vi "SW_Add_Reward_Condition.vi"(8 "error in (no error)":T11, 9 "Main Tree Control in":refnum<vi>, 10 "Calibration parameters":T9={"Timing calibration sw/hw"=1.0, "True FPS"=80.0, "True frame time, s"=0.0125, "Disp. calibration info"=[]} {"True frame time, s" format="%.10g"; "Disp. calibration info"."Speed, µl per ms" format="%.3g"; "True FPS" format="%.10g"; "Timing calibration sw/hw" format="%.10g"}, 11 "Array of conditions in":T8 {"Response"."TTL pulse length, ms" min=0.0 max=10000.0 step=10.0; "Specifier(s)"."Validity criteria(s)"."Validity value" min=0.0 step=0.1 format="%.2g"; "Specifier(s)"."Value" step=1.0 format="%#.2g"}) -> (0 "error out":T11, 3 "Array of conditions out":T8 {"Response"."TTL pulse length, ms" min=0.0 max=10000.0 step=10.0; "Specifier(s)"."Validity criteria(s)"."Validity value" min=0.0 step=0.1 format="%.2g"; "Specifier(s)"."Value" step=1.0 format="%#.2g"})   [LabVIEW 2018, in "Tracker.lvlib"]
uses:
  Tracker.lvlib
  Controls/CTL_Conditions_Array.ctl
  Controls/CTL_Conditions_Cluster.ctl
  Controls/CTL_Condition_type.ctl
  Controls/CTL_Comparison_type.ctl
  Controls/CTL_Validity_check_criteria.ctl
  Controls/CTL_Condition_response_type.ctl
  Controls/CTL_Calibration_parameters.ctl
  Controls/CTL_Dispenser_calibration_info.ctl
  <vilib>/Utility/miscctls.llb/LVPointTypeDef.ctl
panel:
  in  "Save SubCondition":bool
  out "Validity criteria(s)":T2(array[cluster])
  out "Subcondition":T3={"Enabled"=FALSE, "Name"="", "Specifier(s)"=[], "Response"={"Response type"=enum."Air puff", "TTL port"=enum."TTL", "TTL pulse length, ms"=0.0}} caption="Condition" {"Specifier(s)"."Validity criteria(s)"."Validity value" min=0.0 step=0.1 format="%.2g"; "Specifier(s)"."Value" step=1.0 format="%#.2g"}
  in  "TTL pulse length":dbl caption="Disp. volume, ul"
  in  "TTL port":enum16{"TTL"}(ring)
  in  "Response type":T6=enum."Air puff"
  in  "Valid for, units":dbl caption="Has been True for, units" format="%.2g"
  in  "Validity Enabled":bool caption="Enabled"
  in  "SC. Validity Criteria":T1 caption="Validity Criteria"
  in  "Compare against":dbl
  in  "Comparison type":T5
  in  "SubCondition type":T4
  in  "Specifier Enabled":bool caption="Enabled"
  in  "Subcondition #":i32(slide)=5 min=1 max=5 step=1 scale=5.0..1.0
  in  "Specifier(s)":T7(array[cluster])
  in  "C. Name":string caption="Condition Name"
  out "N conditions":i32
  in  "C. Enabled":bool caption="Enabled"
  out "Selected SubCondition":string
  out "Selected Condition":string
  out "Review changes before save":string(tree) caption="Reward and stimulation out"
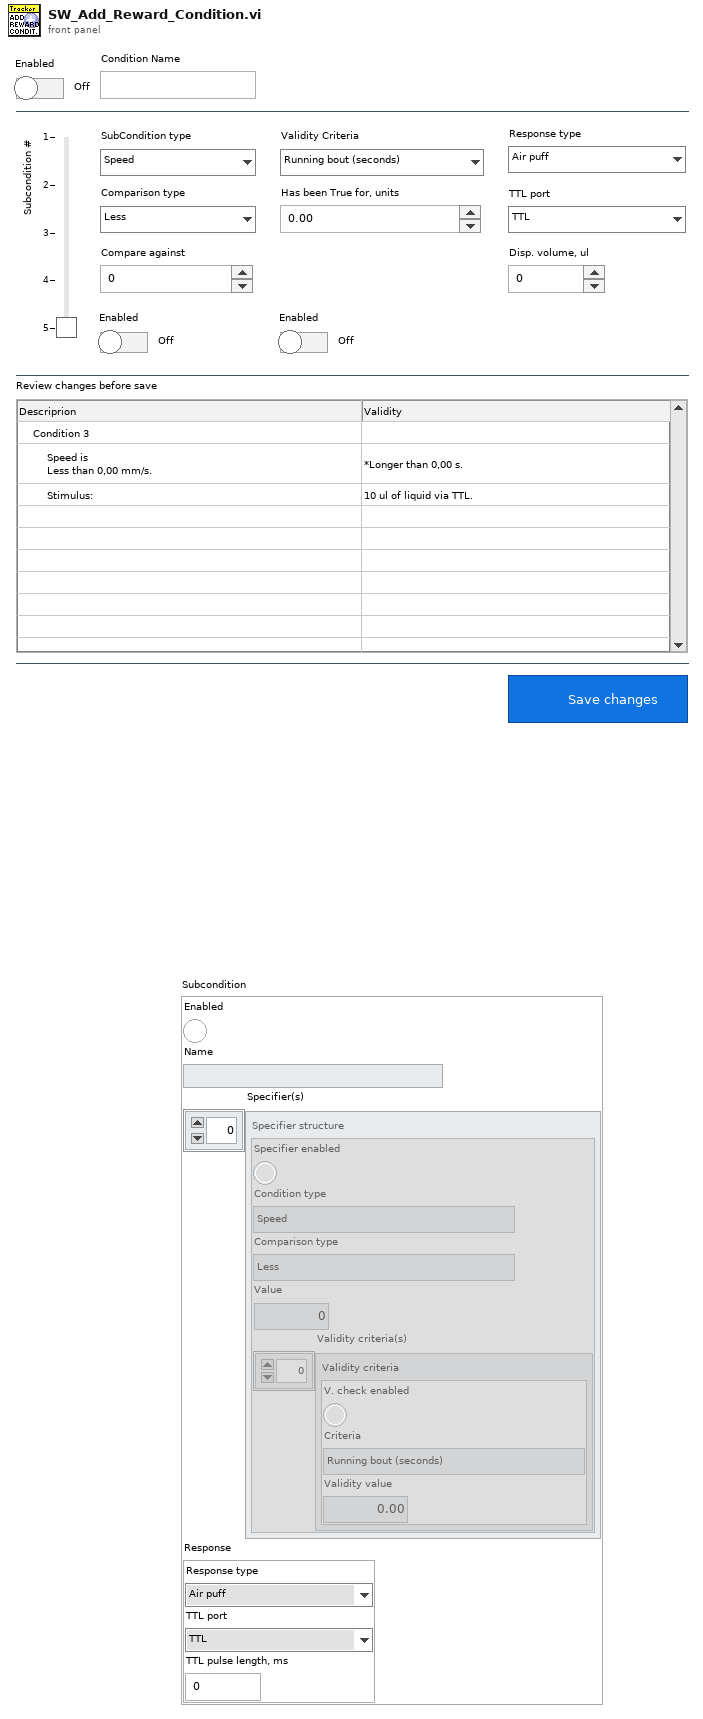
[diagram p1: front panel]
types:
  T1 = typedef "Tracker.lvlib/CTL_Validity_check_criteria.ctl" = enum16{"Running bout (seconds)", "Running bout (meters)"}
  T2 = cluster{"V. check enabled":bool, "Criteria":T1, "Validity value":dbl}[]
  T3 = typedef "Tracker.lvlib/CTL_Conditions_Cluster.ctl" = cluster{"Enabled":bool, "Name":string, "Specifier(s)":cluster{"Specifier enabled":bool, "Condition type":T4, "Comparison type":T5, "Value":dbl, "Validity criteria(s)":cluster{"V. check enabled":bool, "Criteria":T1, "Validity value":dbl}[]}[], "Response":cluster{"Response type":T6, "TTL port":enum16{"TTL"}, "TTL pulse length, ms":dbl}}
  T4 = typedef "Tracker.lvlib/CTL_Condition_type.ctl" = enum16{"Speed", "Zone", "Angle to wall"}
  T5 = typedef "Tracker.lvlib/CTL_Comparison_type.ctl" = enum16{"Less", "Less or Equal", "Equal", "Greater or Equal", "Greater", "Not Equal"}
  T6 = typedef "Tracker.lvlib/CTL_Condition_response_type.ctl" = enum16{"None", "Air puff", "Liquid reward"}
  T7 = cluster{"Specifier enabled":bool, "Condition type":T4, "Comparison type":T5, "Value":dbl, "Validity criteria(s)":cluster{"V. check enabled":bool, "Criteria":T1, "Validity value":dbl}[]}[]
  T8 = typedef "Tracker.lvlib/CTL_Conditions_Array.ctl" = T3[]
  T9 = typedef "Tracker.lvlib/CTL_Calibration_parameters.ctl" = cluster{"Timing calibration sw/hw":dbl, "True FPS":dbl, "True frame time, s":dbl, "Disp. calibration info":T10}
  T10 = typedef "Tracker.lvlib/CTL_Dispenser_calibration_info.ctl" = cluster{"Channel":u8, "Speed, µl per ms":dbl}[]
  T11 = cluster{"Boolean Round":bool, "code":i32, "source":string}
  T12 = typedef "LVPointTypeDef.ctl" = cluster{"Horizontal":i16, "Vertical":i16}
  T13 = cluster{"Response type":T6, "TTL port":enum16{"TTL"}, "TTL pulse length, ms":dbl}
  T14 = cluster{"Specifier enabled":bool, "Condition type":T4, "Comparison type":T5, "Value":dbl, "Validity criteria(s)":cluster{"V. check enabled":bool, "Criteria":T1, "Validity value":dbl}[]}
  T15 = cluster{"V. check enabled":bool, "Criteria":T1, "Validity value":dbl}
  T16 = cluster{"Validity Enabled":bool, "SC. Validity Criteria":T1, "Valid for, units":dbl}
  T17 = cluster{"Response type":T6, "TTL port":enum16{"TTL"}, "TTL pulse length, ms out":dbl}
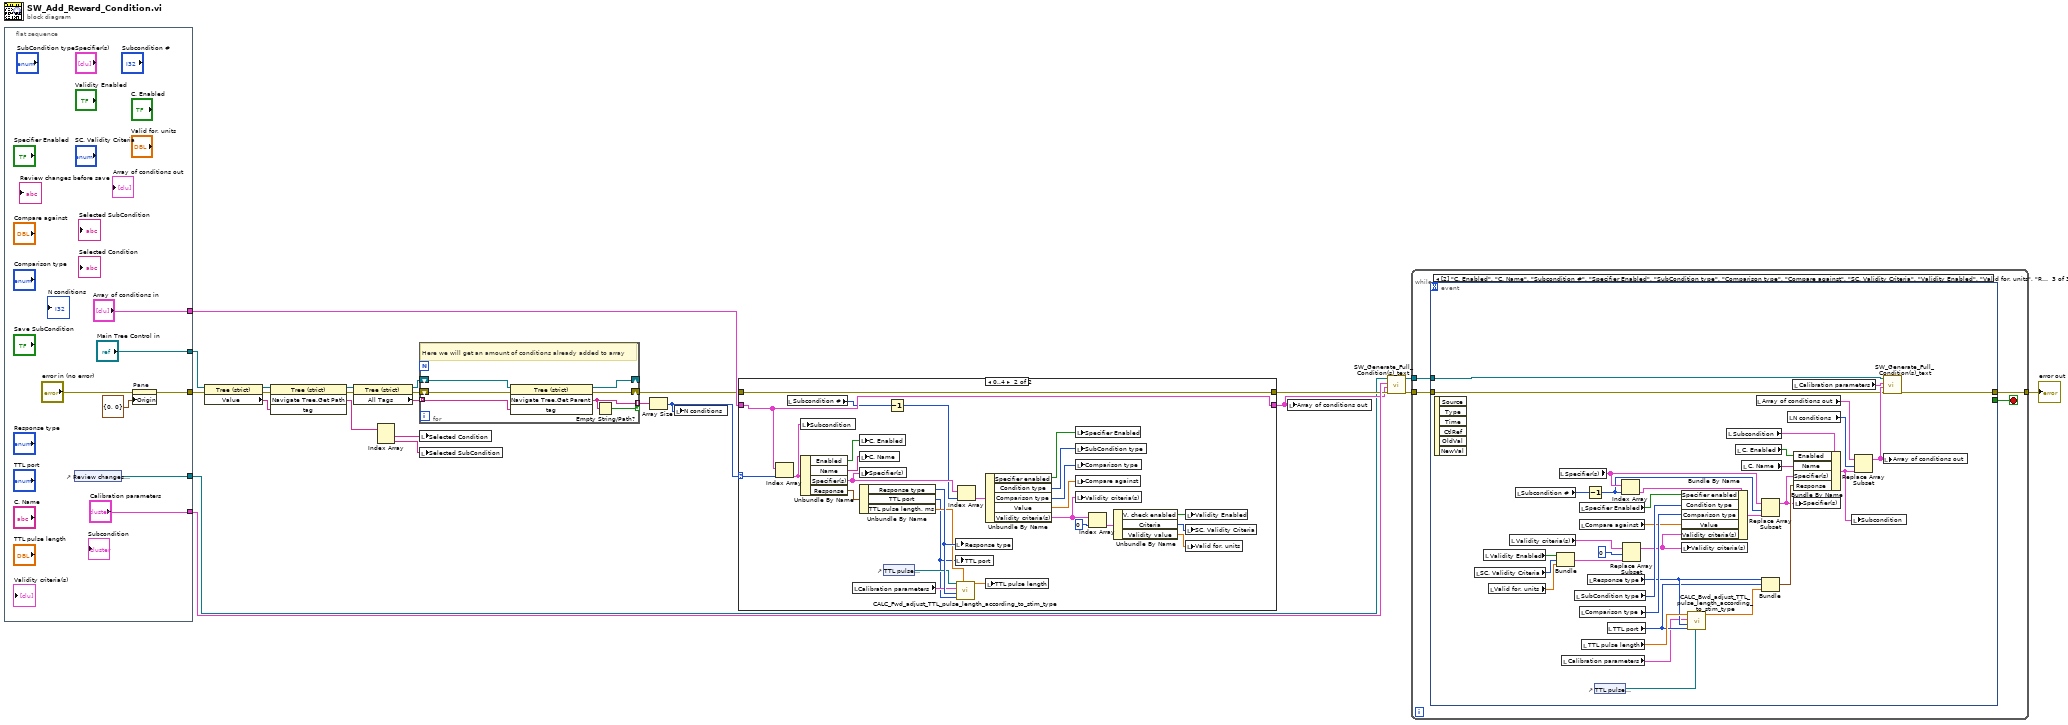
[diagram p0: block diagram]
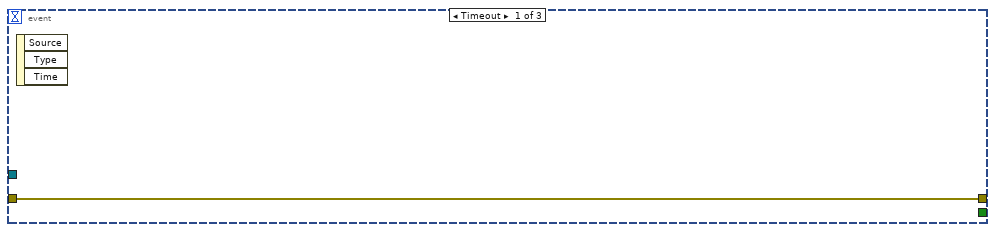
[diagram p2: hidden frame]
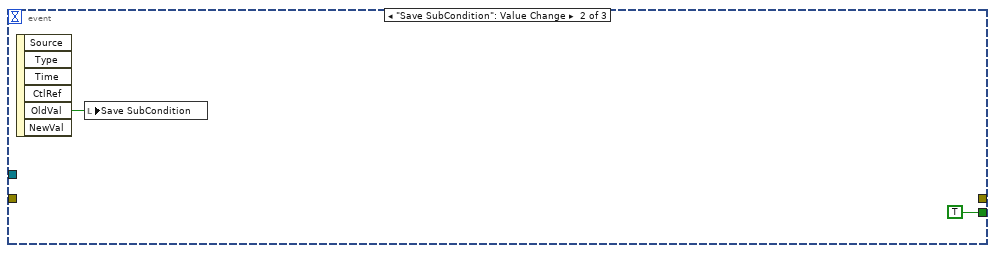
[diagram p3: hidden frame]
diagram:
  n1 = flat-sequence {
    tunnel: [w31] -> w13
    tunnel: [w28] -> w2
    tunnel: ["Main Tree Control in"] -> w24
    tunnel: ["Array of conditions in"] -> w15
    tunnel: ["Calibration parameters"] -> w14
    frame #0 {
      n2 = control-ref of="Review changes before save"() -> (w28:refnum<vi>)
      n3 = property on="Pane" class="Pane"(error in="error in (no error)", "Origin"=T12 {"Horizontal"=0, "Vertical"=0}) -> (error out=w31:errorcluster)  [unwired: 1 in, 1 out]
    }
  }
  n4 = property class="Tree (strict)"(reference=w24, error in=w13) -> (reference out=w22:refnum<vi>, error out=w23:errorcluster, "Value"=w21:string)
  n5 = invoke class="Tree (strict)" method="Navigate Tree.Get Path"(reference=w22, error in=w23, "tag"=w21) -> (reference out=w19:refnum<vi>, error out=w12:errorcluster, "Navigate Tree:Get Path"=w20:string[])  [unwired: 1 in, 1 out]
  n6 = property class="Tree (strict)"(reference=w19, error in=w12) -> (reference out=w18:refnum<vi>, error out=w11:errorcluster, "All Tags"=w17:string[])
  n7 = Index Array(array=w20) -> (element #1=w9:string, element #2=w10:string)  [unwired: 2 in]
  n8 = for {
    tunnel: w17 -> [w37] mode=indexing
    tunnel: [w36] -> w16 mode=indexing if=w35
    shift-right: [w32] -> w7
    shift-left: w11 -> [w34]
    shift-right: [w33] -> _
    shift-left: w18 -> [w38]
    # "Here we will get an amount of conditions already added to array"
    n9 = invoke class="Tree (strict)" method="Navigate Tree.Get Parent"(reference=w38, error in=w34, "tag"=w37) -> (reference out=w33:refnum<vi>, error out=w32:errorcluster, "Navigate Tree:Get Parent"=w36:string)  [unwired: 1 in, 1 out]
    n10 = Empty String/Path?(string/path=w36) -> (empty?=w35:bool)
  }
  n11 = local write "Selected Condition"(w9) -> ()
  n12 = local write "Selected SubCondition"(w10) -> ()
  n13 = Array Size(array=w16) -> (size(s)=w3:i32)
  n14 = local write "N conditions"(w3) -> ()
  n15 = case shown="0..4" w3 {
    selector: w3 -> [_ w67]
    tunnel: w15 -> [w40 w64]
    tunnel: [w40 w64] -> w4
    tunnel: w7 -> [w39 w49]
    tunnel: [w39 w49] -> w8
    frame 5.., Default {
    }
    frame 0..4 {
      n16 = Index Array(array=w64, index=w67) -> (element=w48:T3)
      n17 = local read "Subcondition #"() -> (w62:i32)
      n18 = local write "Subcondition"(w48) -> ()
      n19 = Unbundle By Name(w48) -> ("Enabled"=w66:bool, "Name"=w65:string, "Specifier(s)"=w63:T7, "Response"=w50:T13)
      n20 = local read "Calibration parameters"() -> (w43:T9)
      n21 = local write "C. Enabled"(w66) -> ()
      n22 = local write "C. Name"(w65) -> ()
      n23 = local write "Specifier(s)"(w63) -> ()
      n24 = Unbundle By Name(w50) -> ("Response type"=w46:T6, "TTL port"=w41:enum16{"TTL"}, "TTL pulse length, ms"=w44:dbl)
      n25 = control-ref of="TTL pulse length"() -> (w42:refnum<vi>)
      n26 = Decrement(x=w62) -> (x-1=w61:i32)
      n27 = local write "Response type"(w46) -> ()
      n28 = local write "TTL port"(w41) -> ()
      n29 = call "CALC_Fwd_adjust_TTL_pulse_length_according_to_stim_type.vi"("TTL pulse length, ms in"=w44, "TTL port"=w41, "Response type"=w46, "Calibration parameters"=w43, "TTL pulse length ref in"=w42) -> ("TTL pulse length, ms out"=w45:dbl)  [unwired: 6 in]
      n30 = Index Array(array=w63, index=w61) -> (element=w60:T14)
      n31 = Unbundle By Name(w60) -> ("Specifier enabled"=w59:bool, "Condition type"=w56:T4, "Comparison type"=w57:T5, "Value"=w58:dbl, "Validity criteria(s)"=w47:T2)
      n32 = local write "TTL pulse length"(w45) -> ()
      n33 = local write "Specifier Enabled"(w59) -> ()
      n34 = local write "SubCondition type"(w56) -> ()
      n35 = local write "Comparison type"(w57) -> ()
      n36 = local write "Compare against"(w58) -> ()
      n37 = local write "Validity criteria(s)"(w47) -> ()
      n38 = Index Array(array=w47, index=0) -> (element=w54:T15)
      n39 = Unbundle By Name(w54) -> ("V. check enabled"=w53:bool, "Criteria"=w51:T1, "Validity value"=w52:dbl)
      n40 = local write "Validity Enabled"(w53) -> ()
      n41 = local write "SC. Validity Criteria"(w51) -> ()
      n42 = local write "Valid for, units"(w52) -> ()
    }
  }
  n43 = local write "Array of conditions out"(w4) -> ()
  n44 = call "SW_Generate_Full_Condition(s)_text.vi"("error in (no error)"=w8, "Array of conditions in"=w4, "Calibration parameters"=w14, "TreeControl ref in"=w2) -> ("error out"=w6:errorcluster, "TreeControl ref out"=w1:refnum<vi>)  [unwired: 6 in]
  n45 = while {
    tunnel: w6 -> [w71]
    tunnel: [w70] -> w5
    tunnel: w1 -> [w68]
    stop <- w69 stop-if-true
    n46 = event shown="[2] \"C. Enabled\", \"C. Name\", \"Subcondition #\", \"Specifier Enabled\", \"SubCondition type\", \"Comparison type\", \"Compare against\", \"SC. Validity Criteria\", \"Validity Enabled\", \"Valid for, units\", \"Response type\", \"TTL port\", \"TTL pulse length\": Value Change" {
      selector: _ -> [_ _ _]
      dyn-events: _ -> [_ _ _]
      timeout: _ -> [_ _ _]
      tunnel: w71 -> [w72 _ w83]
      tunnel: [w72 _ w82] -> w70
      tunnel: [_ TRUE _] -> w69
      tunnel: w68 -> [_ _ w81]
      event Timeout {
        n47 = event-data() -> ()  [unwired: 1 in, 3 out]
      }
      event "Save SubCondition": Value Change {
        n48 = event-data() -> ("OldVal"=w74:bool)  [unwired: 1 in, 5 out]
        n49 = local write "Save SubCondition"(w74) -> ()
      }
      event "C. Enabled", "C. Name", "Subcondition #", "Specifier Enabled", "Compare against", "Validity Enabled", "Valid for, units", "TTL port", "TTL pulse length": Value Change {
        n50 = event-data() -> ()  [unwired: 1 in, 6 out]
        n51 = local read "SC. Validity Criteria"() -> (w100:T1)
        n52 = local read "Validity Enabled"() -> (w101:bool)
        n53 = local read "Valid for, units"() -> (w99:dbl)
        n54 = local read "Validity criteria(s)"() -> (w103:T2)
        n55 = local read "Subcondition #"() -> (w109:i32)
        n56 = Bundle("Validity Enabled"=w101, "SC. Validity Criteria"=w100, "Valid for, units"=w99) -> (w98:T16)  [unwired: 1 in]
        n57 = local read "Specifier(s)"() -> (w96:T7)
        n58 = local read "Calibration parameters"() -> (w76:T9)
        n59 = local read "SubCondition type"() -> (w106:T4)
        n60 = local read "Specifier Enabled"() -> (w107:bool)
        n61 = local read "Compare against"() -> (w104:dbl)
        n62 = local read "Comparison type"() -> (w105:T5)
        n63 = local read "TTL pulse length"() -> (w80:dbl)
        n64 = Decrement(x=w109) -> (x-1=w95:i32)
        n65 = local read "Response type"() -> (w79:T6)
        n66 = control-ref of="TTL pulse length"() -> (w75:refnum<vi>)
        n67 = local read "TTL port"() -> (w78:enum16{"TTL"})
        n68 = Index Array(array=w96, index=w95) -> (element=w108:T14)
        n69 = Replace Array Subset(array=w103, new element=w98, index=0) -> (w97:T2)
        n70 = Bundle By Name(cluster=w108, "Specifier enabled"=w107, "Condition type"=w106, "Comparison type"=w105, "Value"=w104, "Validity criteria(s)"=w97) -> (w94:T14)
        n71 = local write "Validity criteria(s)"(w97) -> ()
        n72 = call "CALC_Bwd_adjust_TTL_pulse_length_according_to_stim_type.vi"("TTL pulse length ref in"=w75, "TTL port"=w78, "Response type"=w79, "Calibration parameters"=w76, "TTL pulse length, units, in"=w80) -> ("TTL pulse length, ms out"=w77:dbl)  [unwired: 6 in]
        n73 = local read "Subcondition"() -> (w90:T3)
        n74 = local read "C. Enabled"() -> (w91:bool)
        n75 = local read "C. Name"() -> (w92:string)
        n76 = local read "Array of conditions out"() -> (w88:T8)
        n77 = Replace Array Subset(array=w96, new element=w94, index=w95) -> (w89:T7)
        n78 = Bundle("Response type"=w79, "TTL port"=w78, "TTL pulse length, ms out"=w77) -> (w93:T17)  [unwired: 1 in]
        n79 = local read "N conditions"() -> (w87:i32)
        n80 = local read "Calibration parameters"() -> (w84:T9)
        n81 = Bundle By Name(cluster=w90, "Enabled"=w91, "Name"=w92, "Specifier(s)"=w89, "Response"=w93) -> (w86:T3)
        n82 = local write "Specifier(s)"(w89) -> ()
        n83 = local write "Subcondition"(w86) -> ()
        n84 = Replace Array Subset(array=w88, new element=w86, index=w87) -> (w85:T8)
        n85 = call "SW_Generate_Full_Condition(s)_text.vi"("error in (no error)"=w83, "Array of conditions in"=w85, "Calibration parameters"=w84, "TreeControl ref in"=w81) -> ("error out"=w82:errorcluster)  [unwired: 6 in, 1 out]
        n86 = local write "Array of conditions out"(w85) -> ()
      }
    }
  }
  "error out" <- w5
